vi "LoadImageSequence.vi"   [LabVIEW 2010]
uses:
  ImageGen.dll
  Program Files/Meadowlark Optics/Blink 1920 HDMI/SDK/Blink_C_wrapper.dll
panel:
  # "Demonstrates how to load images to the SLM by looping though 2 images 5 times each"
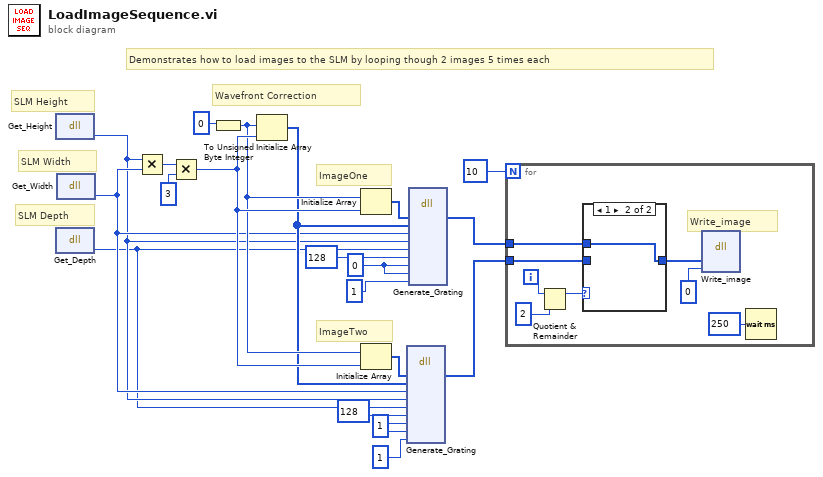
[diagram p0: block diagram]
diagram:
  w15 = 1
  w17 = 0
  # "SLM Depth"
  # "SLM Width"
  # "SLM Height"
  # "ImageTwo"
  # "ImageOne"
  # "Wavefront Correction"
  # "Demonstrates how to load images to the SLM by looping though 2 images 5 times each"
  n1 = dll-call lib="C:/Program Files/Meadowlark Optics/Blink 1920 HDMI/SDK/Blink_C_wrapper.dll" fn="Get_Height"() -> ("return type"=w6:i32)  [unwired: 3 in, 2 out]
  n2 = dll-call lib="C:/Program Files/Meadowlark Optics/Blink 1920 HDMI/SDK/Blink_C_wrapper.dll" fn="Get_Depth"() -> ("return type"=w5:i32)  [unwired: 3 in, 2 out]
  n3 = dll-call lib="C:/Program Files/Meadowlark Optics/Blink 1920 HDMI/SDK/Blink_C_wrapper.dll" fn="Get_Width"() -> ("return type"=w7:i32)  [unwired: 3 in, 2 out]
  n4 = Multiply(x=w6, y=w7) -> (x*y=w13:i32)
  n5 = Multiply(x=w13, y=3) -> (x*y=w11:i32)
  n6 = To Unsigned Byte Integer(number=0) -> (unsigned 8bit integer=w9:u8)
  n7 = Initialize Array(w9, w11) -> (w8:u8[])
  n8 = Initialize Array(w9, w11) -> (w19:u8[])
  n9 = Initialize Array(w9, w11) -> (w16:u8[])
  n10 = dll-call lib="C:/Meadowlark/Repos-git/MeadowlarkBison/BlinkSdkExample/ImageGen.dll" fn="Generate_Grating"("Array"=w16, "WFC"=w8, "Width"=w7, "Height"=w6, "Depth"=w5, "Period"=128, "Increasing"=w15, "Horizontal"=w15, "RGB"=1) -> ("Array"=w3:u8[])  [unwired: 12 in, 2 out]
  n11 = dll-call lib="C:/Meadowlark/Repos-git/MeadowlarkBison/BlinkSdkExample/ImageGen.dll" fn="Generate_Grating"("Array"=w19, "WFC"=w8, "Width"=w7, "Height"=w6, "Depth"=w5, "Period"=128, "Increasing"=w17, "Horizontal"=w17, "RGB"=1) -> ("Array"=w4:u8[])  [unwired: 12 in, 2 out]
  n12 = for {
    N: 10 -> [_]
    tunnel: w4 -> [w23]
    tunnel: w3 -> [w22]
    i -> [w26]
    # "Write_image"
    n13 = Quotient & Remainder(x=w26, y=2) -> (x-y*floor(x/y)=w25:i32)  [unwired: 1 out]
    n14 = case shown="1" w25 {
      tunnel: w23 -> [_ w30]
      tunnel: w22 -> [w29 _]
      tunnel: [w29 w30] -> w21
      frame 0, Default {
      }
      frame 1 {
      }
    }
    n15 = dll-call lib="C:/Program Files/Meadowlark Optics/Blink 1920 HDMI/SDK/Blink_C_wrapper.dll" fn="Write_image"("image_data"=w21, "isEightBit"=0) -> ()  [unwired: 6 in, 2 out]
    n16 = Wait (ms)(milliseconds to wait=u32 250) -> ()  [unwired: 1 out]
  }
